vi "Var-Name-Manipulator-for-ODE-plots-23032016.vi"(5 "In_Rest_Sp_IDs":string[](array[string]), 7 "In_Ex_Mod_IDs":string[](array[string])=["LacI", "TetR"], 8 "error in (no error)":errorcluster, 9 "In_ODE":string[](array[string])=["-(kd*CI)+10*((ko__P1*ng__P1*Ko__P1*RNAP)/(1+Ko__P1*RNAP+(Kr__LacI_P1*LacI)^nc__LacI_P1))+10*((ko__P2*ng__P2*Ko__P2*RNAP)/(1+Ko__P2*RNAP+(Kr__TetR_P2*TetR)^nc__TetR_P2))", "-(kd*GFP)+10*((ko__Promoter_GFP*ng__Promoter_GFP*Ko__Promoter_GFP*RNAP)/(1+Ko__Promoter_GFP*RNAP+(Kr__CI_Promoter_GFP*CI)^nc__CI_Promoter_GFP))"], 10 "In_Tot_Param":string[](array[string])=["ko_r", "nr", "np", "kr_r", "ka_f", "kecdiff", "ko", "kmdiff_f", "kecd", "kc_r", "kr_f", "ka_r", "nc", "kao_r", "kd", "kb", "ng", "ka", "kao_f", "kmdiff_r", "ko_f", "kc_f", "High", "HighTime", "HighTime2", "kd", "kd", "kd", "kd", "RNAP", "ng__P1", "Ko__P1", "ko__P1", "nc__LacI_P1", "Kr__LacI_P1", "RNAP", "ng__P2", "Ko__P2", "ko__P2", "nc__TetR_P2", "Kr__TetR_P2", "RNAP", "ng__Promoter_GFP", "Ko__Promoter_GFP", "ko__Promoter_GFP", "nc__CI_Promoter_GFP", "Kr__CI_Promoter_GFP"], 11 "In_X_for_ODE":string[](array[string])=["CI", "GFP"]) -> (0 "error out":errorcluster, 1 "Out_ODE":string[](array[string]), 2 "Out_Tot_Param":string[](array[string]), 3 "Out_X_for_ODE":string[](array[string]), 4 "Out_Rest_Sp_IDs":string[](array[string]), 6 "Out_Ex_Mod_IDs":string[](array[string]))   [LabVIEW 2014]
doc: "This VI manipulates the variable and parameters name according to the format acceptable to LabVIEW ODE VI.\n\nDesigned By: HB\nhaba@dtu.dk"
uses:
  <vilib>/regexp/Match Regular Expression.xnode
panel:
  out "L-Op":string
  out "R-Op":string
  out "ODE":string[][](table)
  out "Parameters":string[][](table)
  out "X Variables":string[][](table)
  out "Cnt_digit":i32
  out "Cnt_Char":i32
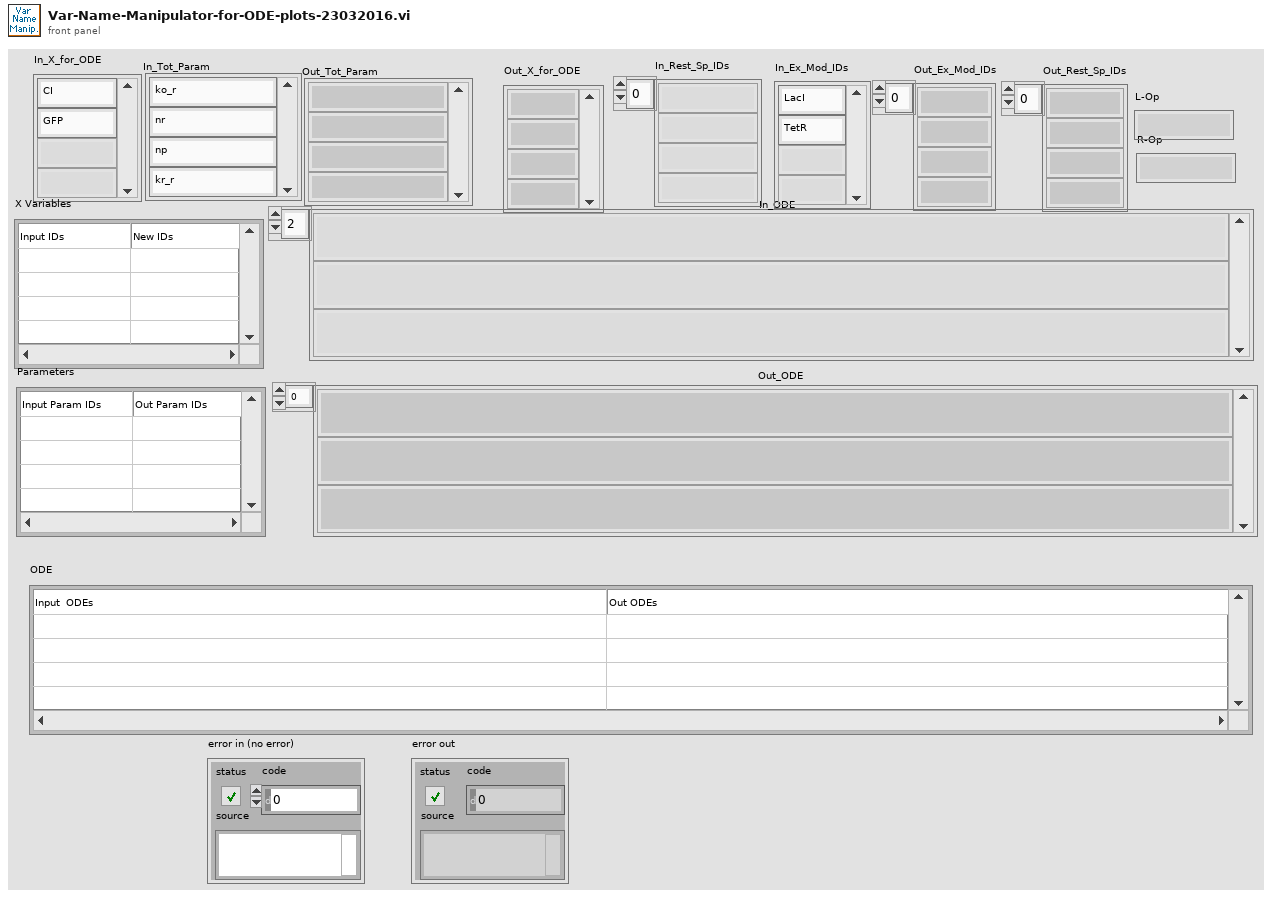
[diagram p1: front panel]
types:
  T1 = enum16{"big-endian, network order", "native, host order", "little-endian"}
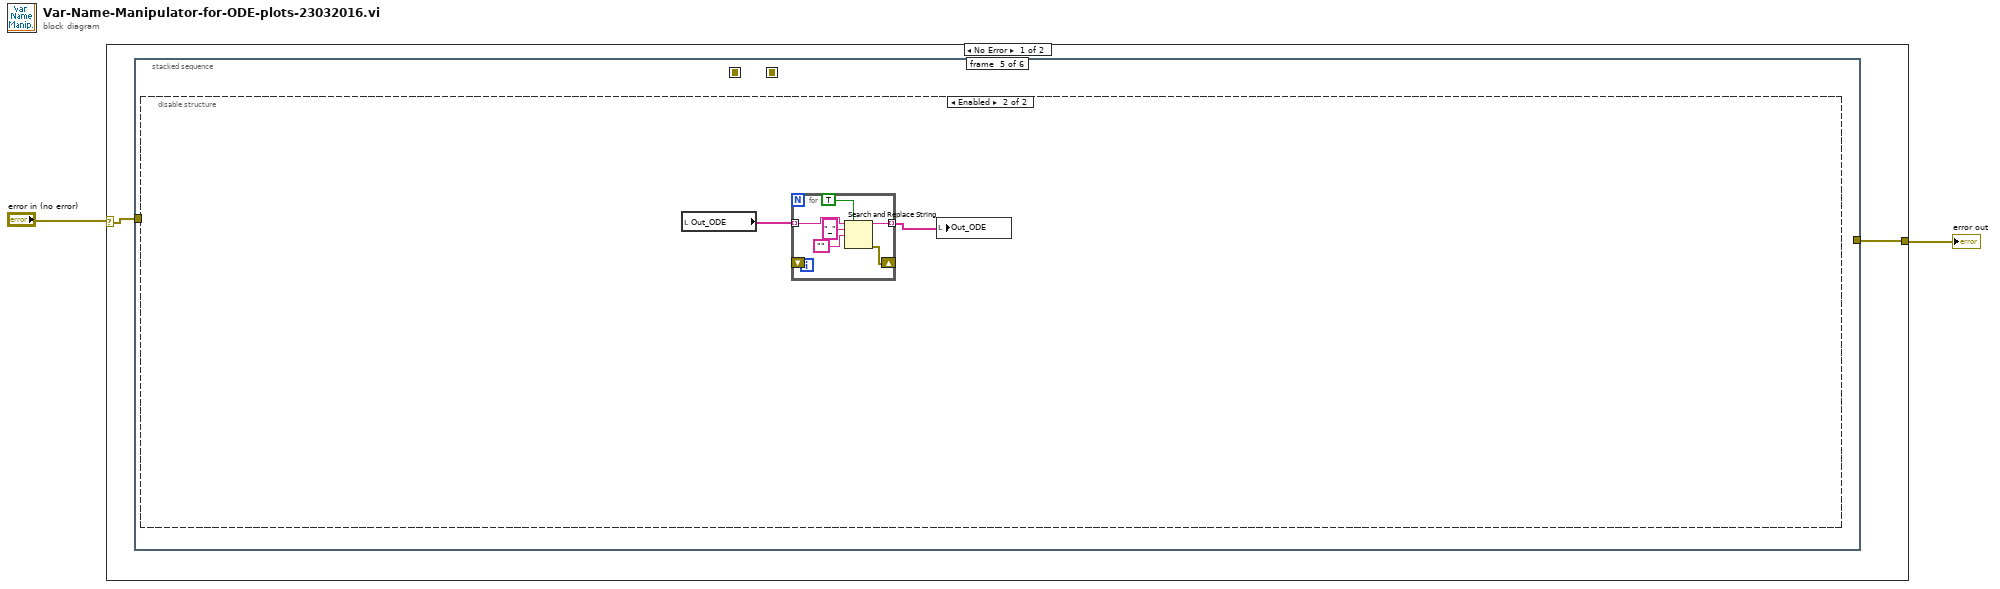
[diagram p0: block diagram]
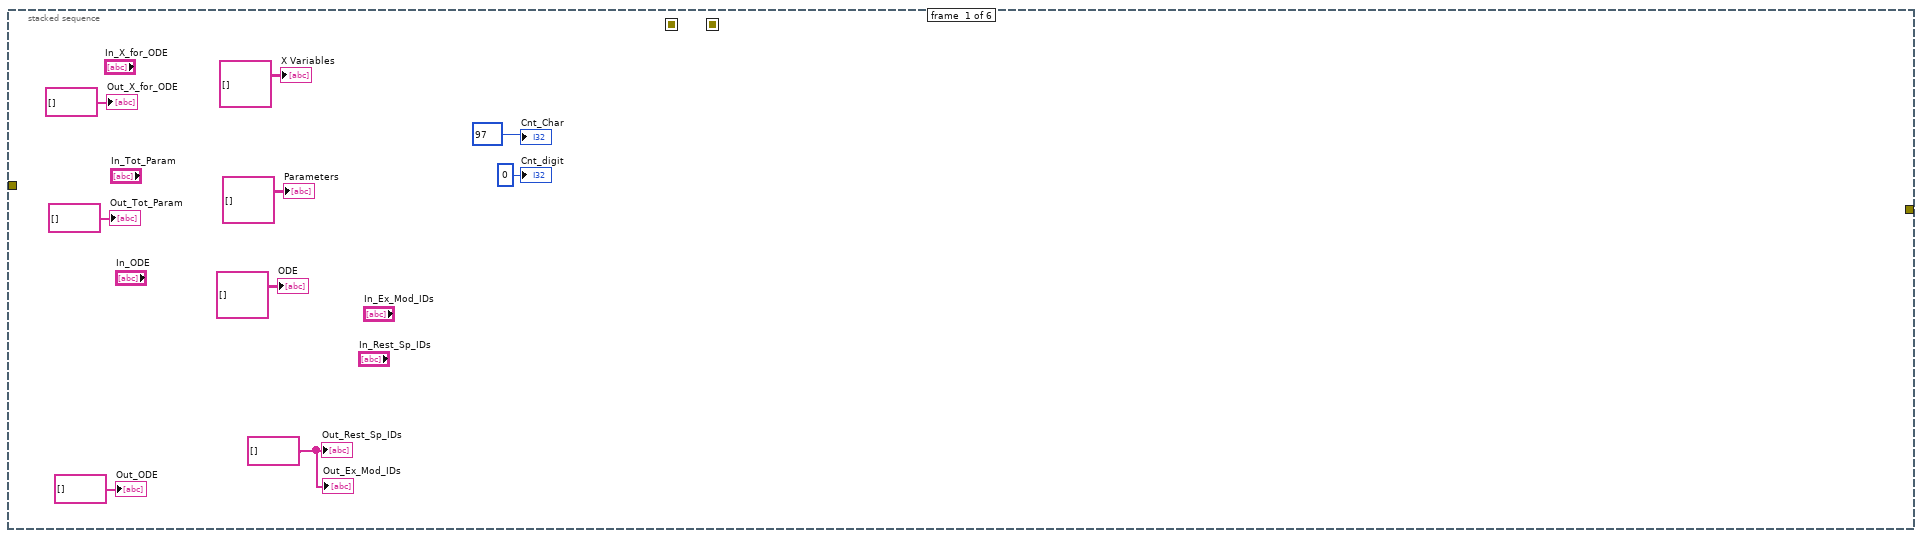
[diagram p2: hidden frame]
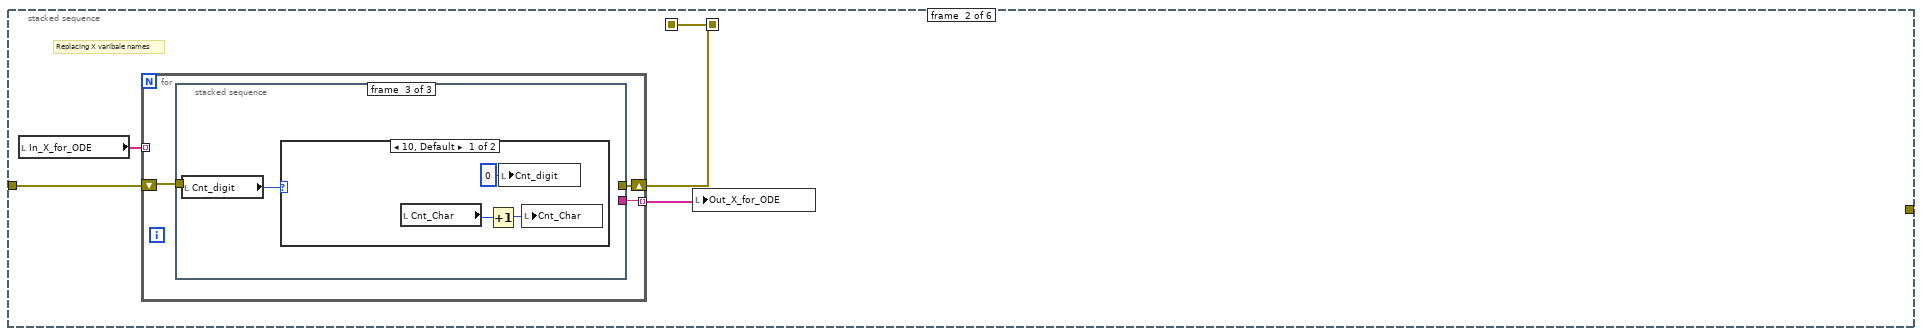
[diagram p3: hidden frame]
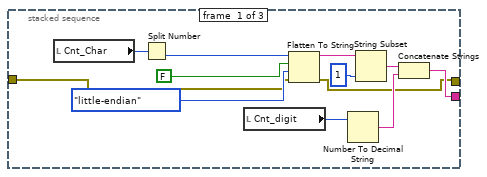
[diagram p4: hidden frame]
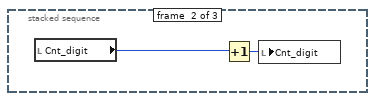
[diagram p5: hidden frame]
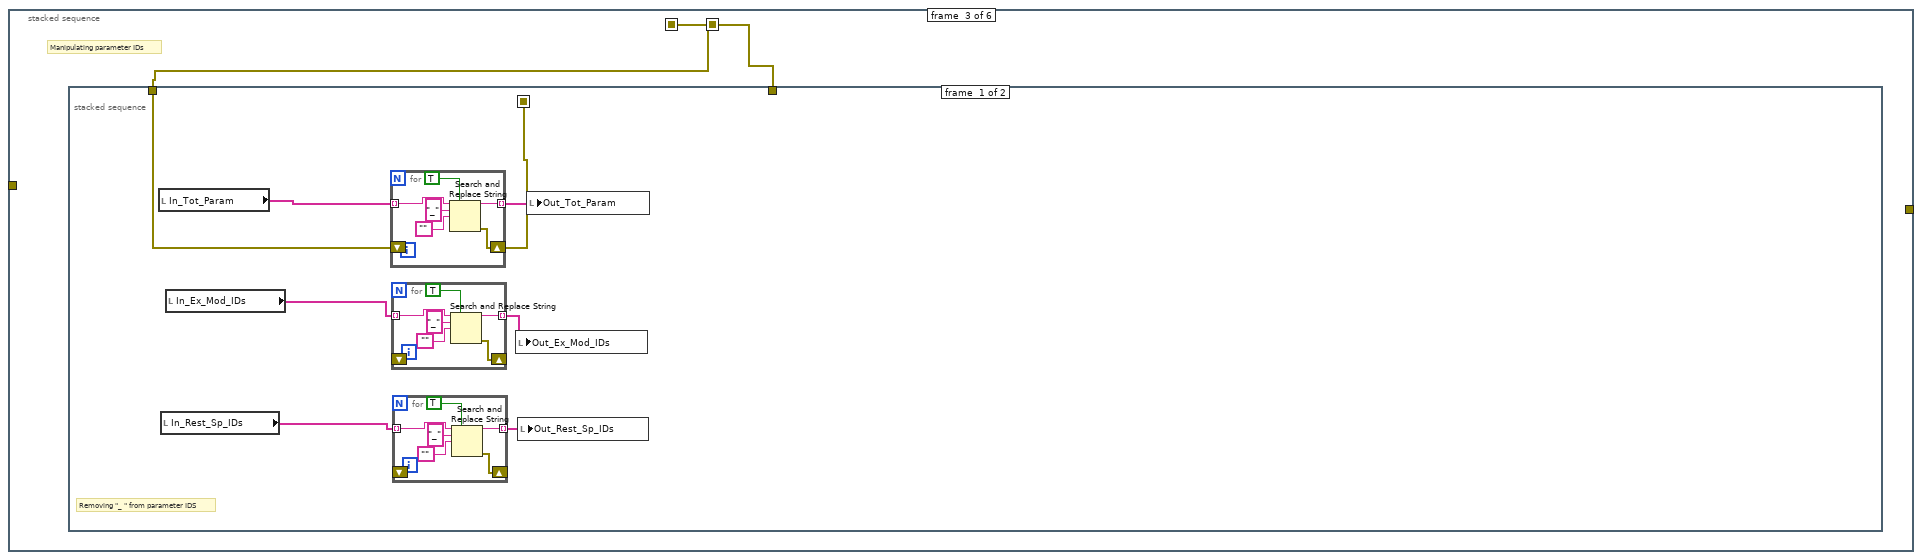
[diagram p7: hidden frame]
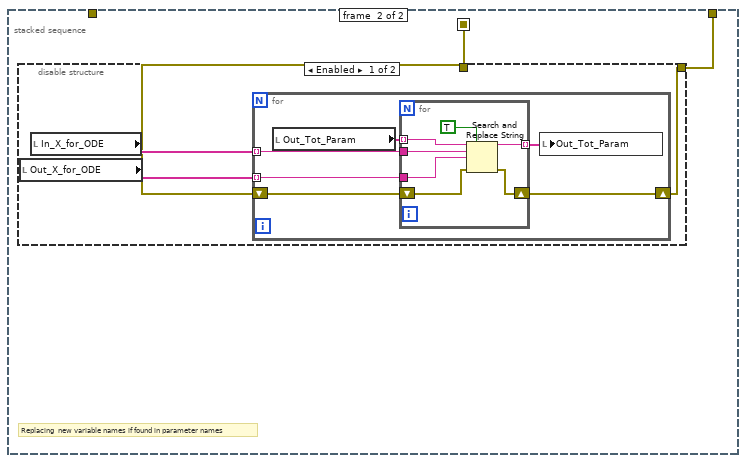
[diagram p8: hidden frame]
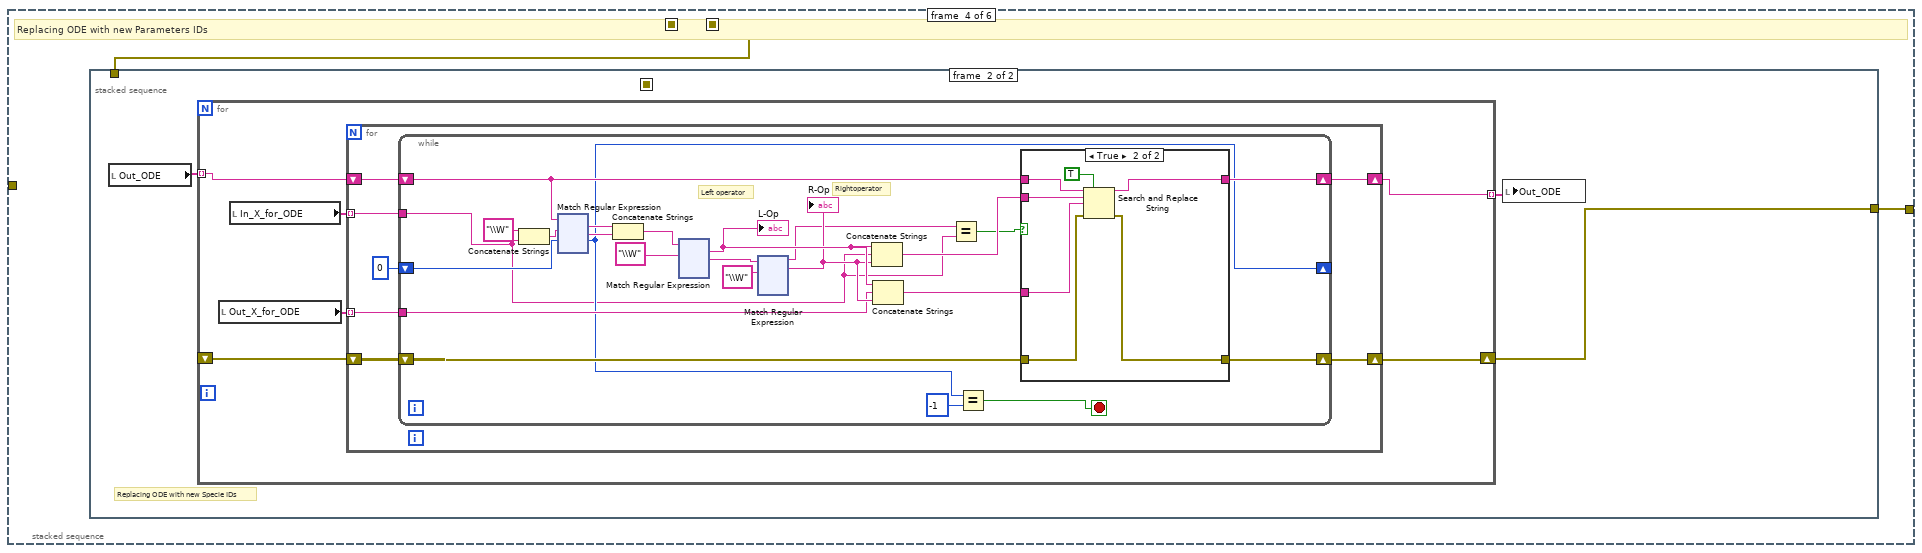
[diagram p10: hidden frame]
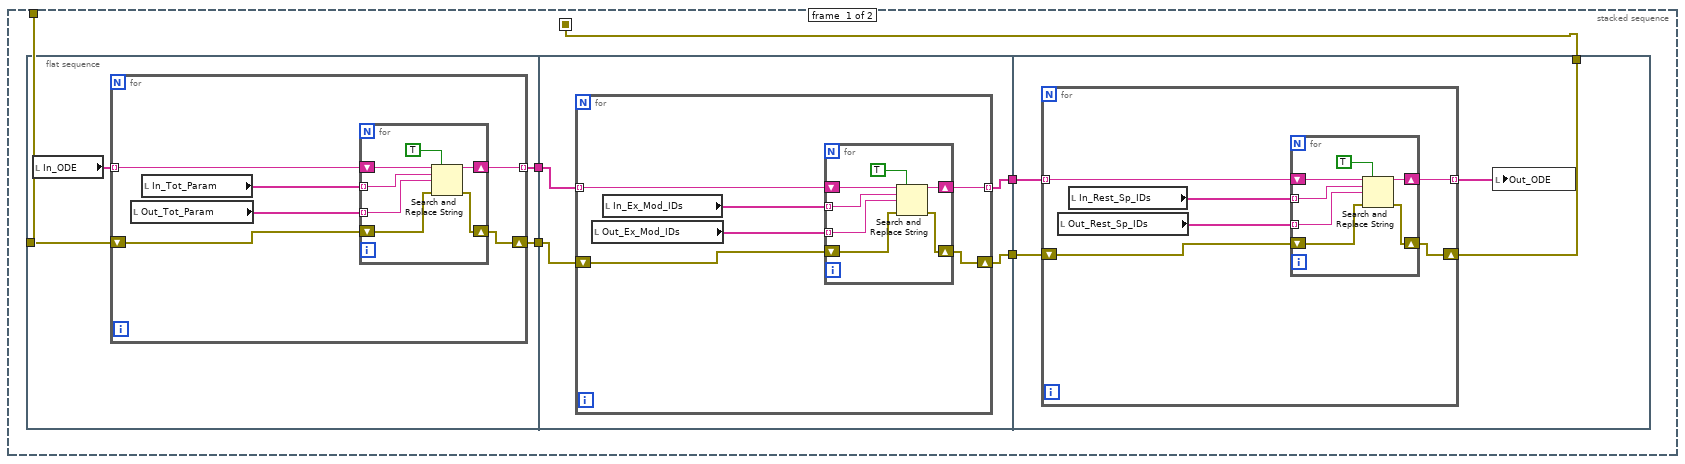
[diagram p11: hidden frame]
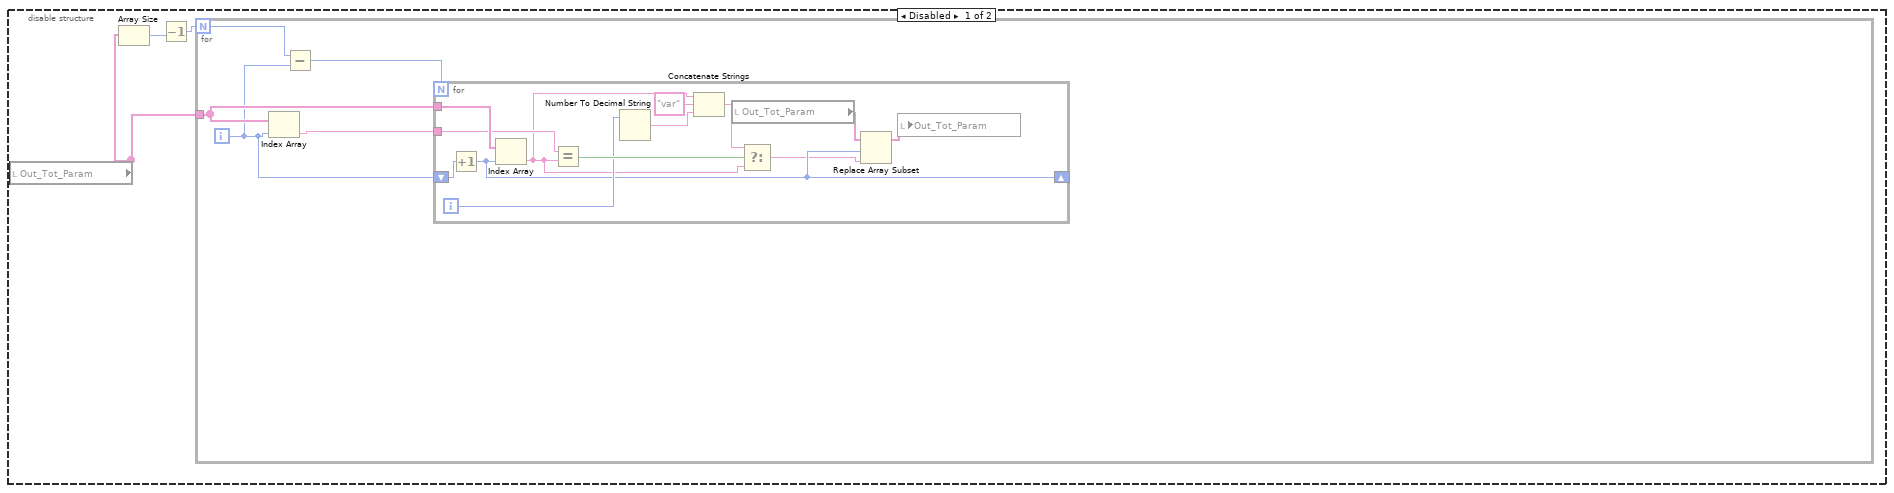
[diagram p13: hidden frame]
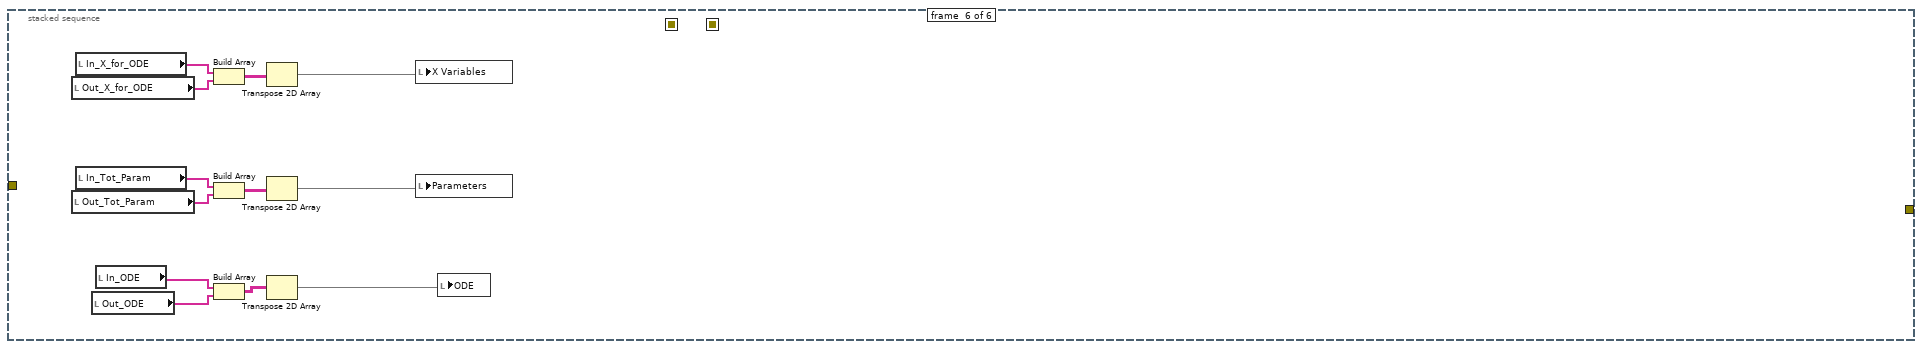
[diagram p14: hidden frame]
diagram:
  n1 = case shown="No Error" "error in (no error)" {
    selector: "error in (no error)" -> [w4 w578]
    tunnel: [w3 w578] -> w1
    frame No Error {
      n2 = stacked-sequence {
        seq-local: [_ w14 _ _ _ _] -> [_ _ w40 _ _ _]
        seq-local: [_ _ w39 _ _ _] -> [_ _ _ w88 _ _]
        tunnel: w4 -> [_ w15 _ _ _ _]
        tunnel: [_ _ _ w87 _ _] -> w3
        frame #0 {
          w5 = string[] [] ("X_Replaced_with")
          "Out_X_for_ODE" <- string[] [] ("X_Replaced_with")
          "Cnt_Char" <- 97
          "Cnt_digit" <- 0 ("Cnt_digit")
          "Out_Tot_Param" <- string[] [] ("Param_Replaced_with")
          "Out_ODE" <- string[] [] ("Out_ODe")
          "X Variables" <- string[][] [] ("X Variables")
          "Parameters" <- string[][] [] ("X Variables")
          "ODE" <- string[][] [] ("X Variables")
          "Out_Rest_Sp_IDs" <- w5
          "Out_Ex_Mod_IDs" <- w5
        }
        frame #1 {
          # "Replacing X varibale names"
          n3 = local read "In_X_for_ODE"() -> (w17:string[])
          n4 = for {
            tunnel: w17 -> [_] mode=indexing
            tunnel: [w20] -> w16 mode=indexing
            shift-right: [w18] -> w14
            shift-left: w15 -> [w19]
            n5 = stacked-sequence {
              tunnel: [w23 _ _] -> w20
              tunnel: w19 -> [w22 _ _]
              tunnel: [w21 _ _] -> w18
              frame #0 {
                n6 = local read "Cnt_Char"() -> (w29:i32)
                n7 = Split Number(x=w29) -> (lo(x)=w32:u16)  [unwired: 1 out]
                n8 = local read "Cnt_digit"() -> (w28:i32)
                n9 = Flatten To String(anything=w32, prepend array or string size? (T)=FALSE, byte order (0:big-endian, network order)=T1."little-endian", error in (no error)=w22) -> (data string=w26:string, error out=w21:errorcluster)  [unwired: 1 out]
                n10 = Number To Decimal String(number=w28) -> (decimal integer string=w24:string)  [unwired: 1 in]
                n11 = String Subset(string=w26, length (rest)=1 ("length (rest)")) -> (substring=w25:string)  [unwired: 1 in]
                n12 = Concatenate Strings(w25, w24) -> (w23:string)
              }
              frame #1 {
                n13 = local read "Cnt_digit"() -> (w34:i32)
                n14 = Increment(x=w34) -> (x+1=w33:i32)
                n15 = local write "Cnt_digit"(w33) -> ()
              }
              frame #2 {
                n16 = local read "Cnt_digit"() -> (w35:i32)
                n17 = case shown="10, Default" w35 {
                  frame 10, Default {
                    n18 = local read "Cnt_Char"() -> (w37:i32)
                    n19 = Increment(x=w37) -> (x+1=w36:i32)
                    n20 = local write "Cnt_digit"(0 ("Cnt_digit")) -> ()
                    n21 = local write "Cnt_Char"(w36) -> ()
                  }
                  frame 0..9 {
                  }
                }
              }
            }
          }
          n22 = local write "Out_X_for_ODE"(w16) -> ()
        }
        frame #2 {
          # "Manipulating parameter IDs"
          n23 = stacked-sequence {
            seq-local: [w45 _] -> [_ w68]
            tunnel: w40 -> [w46 _]
            tunnel: [_ w67] -> w39
            frame #0 {
              # "Removing \"_ \" from parameter IDS"
              n24 = local read "In_Tot_Param"() -> (w48:string[])
              n25 = local read "In_Rest_Sp_IDs"() -> (w43:string[])
              n26 = local read "In_Ex_Mod_IDs"() -> (w44:string[])
              n27 = for {
                tunnel: w48 -> [w66] mode=indexing
                tunnel: [w63] -> w47 mode=indexing
                shift-right: [w61] -> w45
                shift-left: w46 -> [_]
                n28 = Search and Replace String(replace all?=TRUE ("replace all? (F)"), input string=w66, search string="_", replace string="") -> (result string=w63:string, error out=w61:errorcluster)  [unwired: 4 in, 2 out]
              }
              n29 = for {
                tunnel: w44 -> [w60] mode=indexing
                tunnel: [w57] -> w42 mode=indexing
                shift-right: [w55] -> _
                shift-left: _ -> [_]
                n30 = Search and Replace String(replace all?=TRUE ("replace all? (F)"), input string=w60, search string="_", replace string="") -> (result string=w57:string, error out=w55:errorcluster)  [unwired: 4 in, 2 out]
              }
              n31 = for {
                tunnel: w43 -> [w54] mode=indexing
                tunnel: [w51] -> w41 mode=indexing
                shift-right: [w49] -> _
                shift-left: _ -> [_]
                n32 = Search and Replace String(replace all?=TRUE ("replace all? (F)"), input string=w54, search string="_", replace string="") -> (result string=w51:string, error out=w49:errorcluster)  [unwired: 4 in, 2 out]
              }
              n33 = local write "Out_Ex_Mod_IDs"(w42) -> ()
              n34 = local write "Out_Rest_Sp_IDs"(w41) -> ()
              n35 = local write "Out_Tot_Param"(w47) -> ()
            }
            frame #1 {
              # "Replacing  new variable names if found in parameter names"
              n36 = disable-structure shown="Enabled" {
                disable-tunnel: w68 -> [w70 w86]
                disable-tunnel: [w69 w86] -> w67
                frame Enabled {
                  n37 = local read "Out_X_for_ODE"() -> (w71:string[])
                  n38 = local read "In_X_for_ODE"() -> (w72:string[])
                  n39 = for {
                    tunnel: w72 -> [w75] mode=indexing
                    tunnel: w71 -> [w77] mode=indexing
                    shift-right: [w74] -> w69
                    shift-left: w70 -> [w73]
                    n40 = local read "Out_Tot_Param"() -> (w78:string[])
                    n41 = for {
                      tunnel: w78 -> [w82] mode=indexing
                      tunnel: w77 -> [w85]
                      tunnel: [w83] -> w76 mode=indexing
                      tunnel: w75 -> [w81]
                      shift-right: [w80] -> w74
                      shift-left: w73 -> [w79]
                      n42 = Search and Replace String(replace all?=TRUE ("replace all? (F)"), input string=w82, search string=w81, replace string=w85, error in=w79) -> (result string=w83:string, error out=w80:errorcluster)  [unwired: 3 in, 2 out]
                    }
                    n43 = local write "Out_Tot_Param"(w76) -> ()
                  }
                }
                frame Disabled {
                }
              }
            }
          }
        }
        frame #3 {
          # "Replacing ODE with new Parameters IDs"
          n44 = stacked-sequence {
            seq-local: [w89 _] -> [_ _]
            tunnel: w88 -> [w94 _]
            tunnel: [_ w146] -> w87
            frame #0 {
              n45 = flat-sequence {
                tunnel: w94 -> [w98]
                tunnel: [w96] -> w93
                tunnel: [w95] -> w91
                tunnel: w93 -> [w115]
                tunnel: [w114] -> w92
                tunnel: w91 -> [w113]
                tunnel: [w112] -> w90
                tunnel: w92 -> [w132]
                tunnel: w90 -> [w130]
                tunnel: [w129] -> w89
                frame #0 {
                  n46 = local read "In_ODE"() -> (w97:string[])
                  n47 = for {
                    tunnel: w97 -> [w104] mode=indexing
                    tunnel: [w101] -> w96 mode=indexing
                    shift-right: [w100] -> w95
                    shift-left: w98 -> [w99]
                    n48 = local read "Out_Tot_Param"() -> (w102:string[])
                    n49 = local read "In_Tot_Param"() -> (w103:string[])
                    n50 = for {
                      tunnel: w103 -> [w110] mode=indexing
                      tunnel: w102 -> [w109] mode=indexing
                      shift-right: [w107] -> w101
                      shift-left: w104 -> [w111]
                      shift-right: [w106] -> w100
                      shift-left: w99 -> [w105]
                      n51 = Search and Replace String(replace all?=TRUE ("replace all? (F)"), input string=w111, search string=w110, replace string=w109, error in=w105) -> (result string=w107:string, error out=w106:errorcluster)  [unwired: 3 in, 2 out]
                    }
                  }
                }
                frame #1 {
                  n52 = for {
                    tunnel: w115 -> [w121] mode=indexing
                    tunnel: [w118] -> w114 mode=indexing
                    shift-right: [w117] -> w112
                    shift-left: w113 -> [w116]
                    n53 = local read "Out_Ex_Mod_IDs"() -> (w119:string[])
                    n54 = local read "In_Ex_Mod_IDs"() -> (w120:string[])
                    n55 = for {
                      tunnel: w120 -> [w127] mode=indexing
                      tunnel: w119 -> [w126] mode=indexing
                      shift-right: [w124] -> w118
                      shift-left: w121 -> [w128]
                      shift-right: [w123] -> w117
                      shift-left: w116 -> [w122]
                      n56 = Search and Replace String(replace all?=TRUE ("replace all? (F)"), input string=w128, search string=w127, replace string=w126, error in=w122) -> (result string=w124:string, error out=w123:errorcluster)  [unwired: 3 in, 2 out]
                    }
                  }
                }
                frame #2 {
                  n57 = for {
                    tunnel: w132 -> [w138] mode=indexing
                    tunnel: [w135] -> w131 mode=indexing
                    shift-right: [w134] -> w129
                    shift-left: w130 -> [w133]
                    n58 = local read "Out_Rest_Sp_IDs"() -> (w136:string[])
                    n59 = local read "In_Rest_Sp_IDs"() -> (w137:string[])
                    n60 = for {
                      tunnel: w137 -> [w144] mode=indexing
                      tunnel: w136 -> [w143] mode=indexing
                      shift-right: [w141] -> w135
                      shift-left: w138 -> [w145]
                      shift-right: [w140] -> w134
                      shift-left: w133 -> [w139]
                      n61 = Search and Replace String(replace all?=TRUE ("replace all? (F)"), input string=w145, search string=w144, replace string=w143, error in=w139) -> (result string=w141:string, error out=w140:errorcluster)  [unwired: 3 in, 2 out]
                    }
                  }
                  n62 = local write "Out_ODE"(w131) -> ()
                }
              }
            }
            frame #1 {
              # "Replacing ODE with new Specie IDs"
              n63 = local read "Out_ODE"() -> (w148:string[])
              n64 = for {
                tunnel: w148 -> [w154] mode=indexing
                tunnel: [w151] -> w147 mode=indexing
                shift-right: [w150] -> w146
                shift-left: _ -> [w149]
                n65 = local read "Out_X_for_ODE"() -> (w152:string[])
                n66 = local read "In_X_for_ODE"() -> (w153:string[])
                n67 = for {
                  tunnel: w153 -> [w157] mode=indexing
                  tunnel: w152 -> [w156] mode=indexing
                  shift-right: [w161] -> w151
                  shift-left: w154 -> [w158]
                  shift-right: [w159] -> w150
                  shift-left: w149 -> [w160]
                  n68 = while {
                    tunnel: w157 -> [w163]
                    tunnel: w156 -> [w170]
                    shift-right: [w183] -> w159
                    shift-left: w160 -> [w184]
                    shift-right: [w185] -> w161
                    shift-left: w158 -> [w174]
                    shift-right: [w165] -> _
                    shift-left: 0 ("y") -> [w167]
                    stop <- w166 stop-if-true
                    # "Rightoperator"
                    # "Left operator"
                    n69 = Concatenate Strings("\\W" ("regular expression"), w163) -> (w180:string)
                    n70 = xnode "Match Regular Expression"("input string"=w174, "regular expression"=w180, "offset (0)"=w167) -> ("whole match"=w179:string, "after match"=w178:string, "offset past match"=w165:i32)  [unwired: 3 in, 2 out]
                    n71 = Concatenate Strings(w179, w178) -> (w176:string)
                    n72 = xnode "Match Regular Expression"("input string"=w176, "regular expression"="\\W") -> ("whole match"=w172:string, "after match"=w175:string)  [unwired: 4 in, 3 out]
                    "L-Op" <- w172
                    n73 = xnode "Match Regular Expression"("input string"=w175, "regular expression"="\\W") -> ("before match"=w164:string, "whole match"=w171:string)  [unwired: 4 in, 3 out]
                    "R-Op" <- w171
                    n74 = Concatenate Strings(w172, w163, w171) -> (w173:string)
                    n75 = Concatenate Strings(w172, w170, w171) -> (w169:string)
                    n76 = Equal?(x=w164, y=w163) -> (x = y?=w162:bool)
                    n77 = Equal?(x=w165, y=-1) -> (x = y?=w166:bool)
                    n78 = case shown="True" w162 {
                      tunnel: [w187 w193] -> w185
                      tunnel: w184 -> [w186 w192]
                      tunnel: [w186 w191] -> w183
                      tunnel: w174 -> [w187 w190]
                      tunnel: w173 -> [_ w189]
                      tunnel: w169 -> [_ w188]
                      frame False {
                      }
                      frame True {
                        n79 = Search and Replace String(replace all?=TRUE ("replace all? (F)"), input string=w190, search string=w189, replace string=w188, error in=w192) -> (result string=w193:string, error out=w191:errorcluster)  [unwired: 3 in, 2 out]
                      }
                    }
                  }
                }
              }
              n80 = local write "Out_ODE"(w147) -> ()
            }
          }
        }
        frame #4 {
          n81 = disable-structure shown="Enabled" {
            frame Disabled {
              n82 = local read "Out_Tot_Param"() -> (w539:string[])
              n83 = Array Size(array=w539) -> (size(s)=w538:i32)
              n84 = Decrement(x=w538) -> (x-1=w537:i32)
              n85 = for {
                N: w537 -> [w544]
                tunnel: w539 -> [w542]
                i -> [w540]
                n86 = Index Array(array=w542, index=w540) -> (element=w541:string)
                n87 = Subtract(x=w544, y=w540) -> (x-y=w543:i32)
                n88 = for {
                  N: w543 -> [_]
                  tunnel: w542 -> [w557]
                  tunnel: w541 -> [w556]
                  shift-right: [w547] -> _
                  shift-left: w540 -> [w554]
                  i -> [w550]
                  n89 = Increment(x=w554) -> (x+1=w547:i32)
                  n90 = Index Array(array=w557, index=w547) -> (element=w549:string)
                  n91 = Equal?(x=w556, y=w549) -> (x = y?=w555:bool)
                  n92 = Number To Decimal String(number=w550) -> (decimal integer string=w551:string)  [unwired: 1 in]
                  n93 = Concatenate Strings(w549, "var" ("string"), w551) -> (w553:string)
                  n94 = local read "Out_Tot_Param"() -> (w548:string[])
                  n95 = Select(t=w553, s=w555, f=w549) -> (s? t:f=w546:string)
                  n96 = Replace Array Subset(array=w548, new element=w546, index=w547) -> (w545:string[])
                  n97 = local write "Out_Tot_Param"(w545) -> ()
                }
              }
            }
            frame Enabled {
              n98 = local read "Out_ODE"() -> (w559:string[])
              n99 = for {
                tunnel: w559 -> [w565] mode=indexing
                tunnel: [w562] -> w558 mode=indexing
                shift-right: [w560] -> _
                shift-left: _ -> [_]
                n100 = Search and Replace String(replace all?=TRUE ("replace all? (F)"), input string=w565, search string="_", replace string="") -> (result string=w562:string, error out=w560:errorcluster)  [unwired: 4 in, 2 out]
              }
              n101 = local write "Out_ODE"(w558) -> ()
            }
          }
        }
        frame #5 {
          n102 = local read "Out_X_for_ODE"() -> (w575:string[])
          n103 = local read "Out_Tot_Param"() -> (w572:string[])
          n104 = local read "In_X_for_ODE"() -> (w576:string[])
          n105 = local read "In_Tot_Param"() -> (w571:string[])
          n106 = local read "Out_ODE"() -> (w567:string[])
          n107 = local read "In_ODE"() -> (w568:string[])
          n108 = Build Array(w576, w575) -> (w577:string[][])
          n109 = Build Array(w571, w572) -> (w570:string[][])
          n110 = Build Array(w568, w567) -> (w569:string[][])
          n111 = Transpose 2D Array(2D array=w577) -> (transposed array=w574:string[][])
          n112 = Transpose 2D Array(2D array=w570) -> (transposed array=w573:string[][])
          n113 = Transpose 2D Array(2D array=w569) -> (transposed array=w566:string[][])
          n114 = local write "X Variables"(w574) -> ()
          n115 = local write "Parameters"(w573) -> ()
          n116 = local write "ODE"(w566) -> ()
        }
      }
    }
    frame Error {
    }
  }
  "error out" <- w1
